vi "calc_VoltageStepWaveform_v0.03.vi"(0 "New input cluster":T1={"Which Position to use for Experiment"=enum."Jumper Safe Position", "Duration (s)"=0.0, "Delay (s)"=0.0, "Step Width (s)"=0.0, "Voltage Start (mV)"=1.0, "Voltage Step (mV)"=1.0, "Replicates"=1.0, "Voltage End (mV)"=0.0, "Number of Step"=0.0, "Vholding (mV)"=2.0, "Valve 1 Position"=2, "Valve 2 Position"=2, "Valve 3 Position"=2, "valve 1 used now?"=FALSE, "valve 2 used now?"=FALSE, "valve 3 used now? "=TRUE, "Total Step Time (s)"=0.0, "Maintain Final Voltage until end?"=TRUE, "protocol Preview"=[]} {"Valve 3 Position" min=1 max=8; "Valve 2 Position" min=1 max=8; "Valve 1 Position" min=1 max=8}, 1 "Clear Waveform?":bool, 5 "Old input cluster":T1={"Which Position to use for Experiment"=enum."Jumper Safe Position", "Duration (s)"=0.0, "Delay (s)"=0.0, "Step Width (s)"=0.0, "Voltage Start (mV)"=1.0, "Voltage Step (mV)"=1.0, "Replicates"=1.0, "Voltage End (mV)"=0.0, "Number of Step"=0.0, "Vholding (mV)"=2.0, "Valve 1 Position"=2, "Valve 2 Position"=2, "Valve 3 Position"=2, "valve 1 used now?"=FALSE, "valve 2 used now?"=FALSE, "valve 3 used now? "=TRUE, "Total Step Time (s)"=0.0, "Maintain Final Voltage until end?"=TRUE, "protocol Preview"=[]} {"Valve 3 Position" min=1 max=8; "Valve 2 Position" min=1 max=8; "Valve 1 Position" min=1 max=8}, 7 "sample freq":i32=10000, 11 "error in":errorcluster) -> (4 "output cluster":T1={"Which Position to use for Experiment"=enum."Jumper Safe Position", "Duration (s)"=0.0, "Delay (s)"=0.0, "Step Width (s)"=0.0, "Voltage Start (mV)"=1.0, "Voltage Step (mV)"=1.0, "Replicates"=1.0, "Voltage End (mV)"=0.0, "Number of Step"=0.0, "Vholding (mV)"=2.0, "Valve 1 Position"=2, "Valve 2 Position"=2, "Valve 3 Position"=2, "valve 1 used now?"=FALSE, "valve 2 used now?"=FALSE, "valve 3 used now? "=TRUE, "Total Step Time (s)"=0.0, "Maintain Final Voltage until end?"=TRUE, "protocol Preview"=[]} {"Valve 3 Position" min=1 max=8; "Valve 2 Position" min=1 max=8; "Valve 1 Position" min=1 max=8}, 15 "error out":errorcluster)   [LabVIEW 2019]
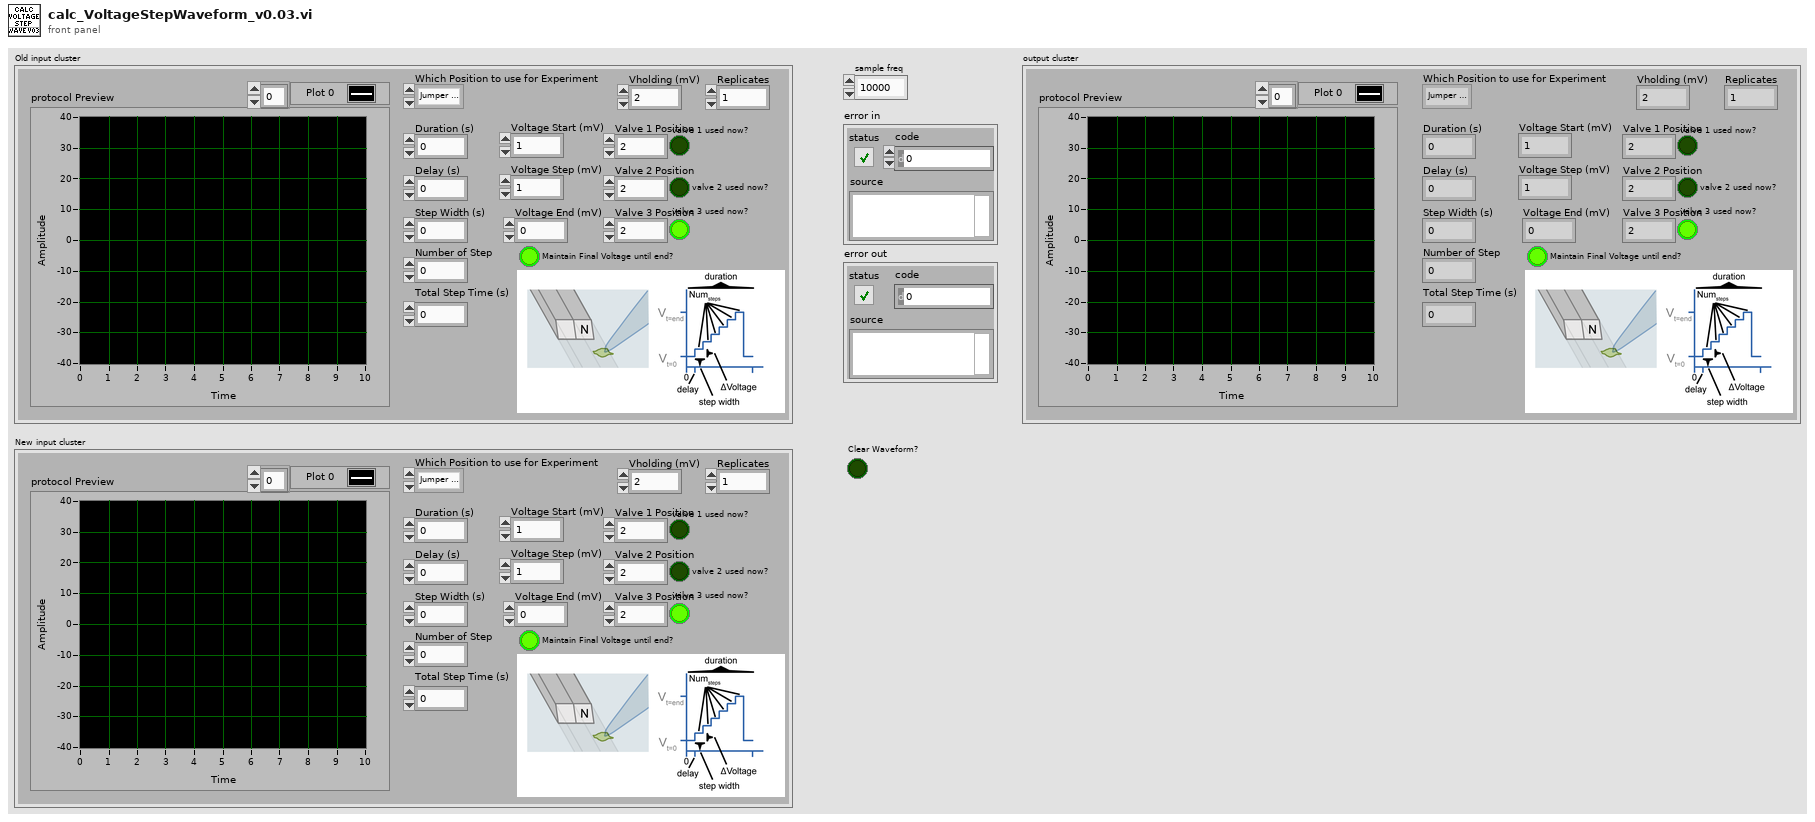
[diagram p1: front panel]
types:
  T1 = cluster{"Which Position to use for Experiment":enum16{"Jumper Safe Position", "Experiment Safe Position", "Jumper Position A", "Jumper Position B", "Jumper Position C", "Jumper Position o-A", "Jumper Position A-o", "Jumper Position A-B", "Jumper Position B-A", "Jumper Position B-C", "Jumper Position C-B", "Jumper Position C-o", "Jumper Position o-C", "Don't Move"}, "Duration (s)":dbl, "Delay (s)":dbl, "Step Width (s)":dbl, "Voltage Start (mV)":dbl, "Voltage Step (mV)":dbl, "Replicates":dbl, "Voltage End (mV)":dbl, "Number of Step":dbl, "Vholding (mV)":dbl, "Valve 1 Position":i16, "Valve 2 Position":i16, "Valve 3 Position":i16, "valve 1 used now?":bool, "valve 2 used now?":bool, "valve 3 used now? ":bool, "Total Step Time (s)":dbl, "Maintain Final Voltage until end?":bool, "protocol Preview":waveform(dbl)[]}
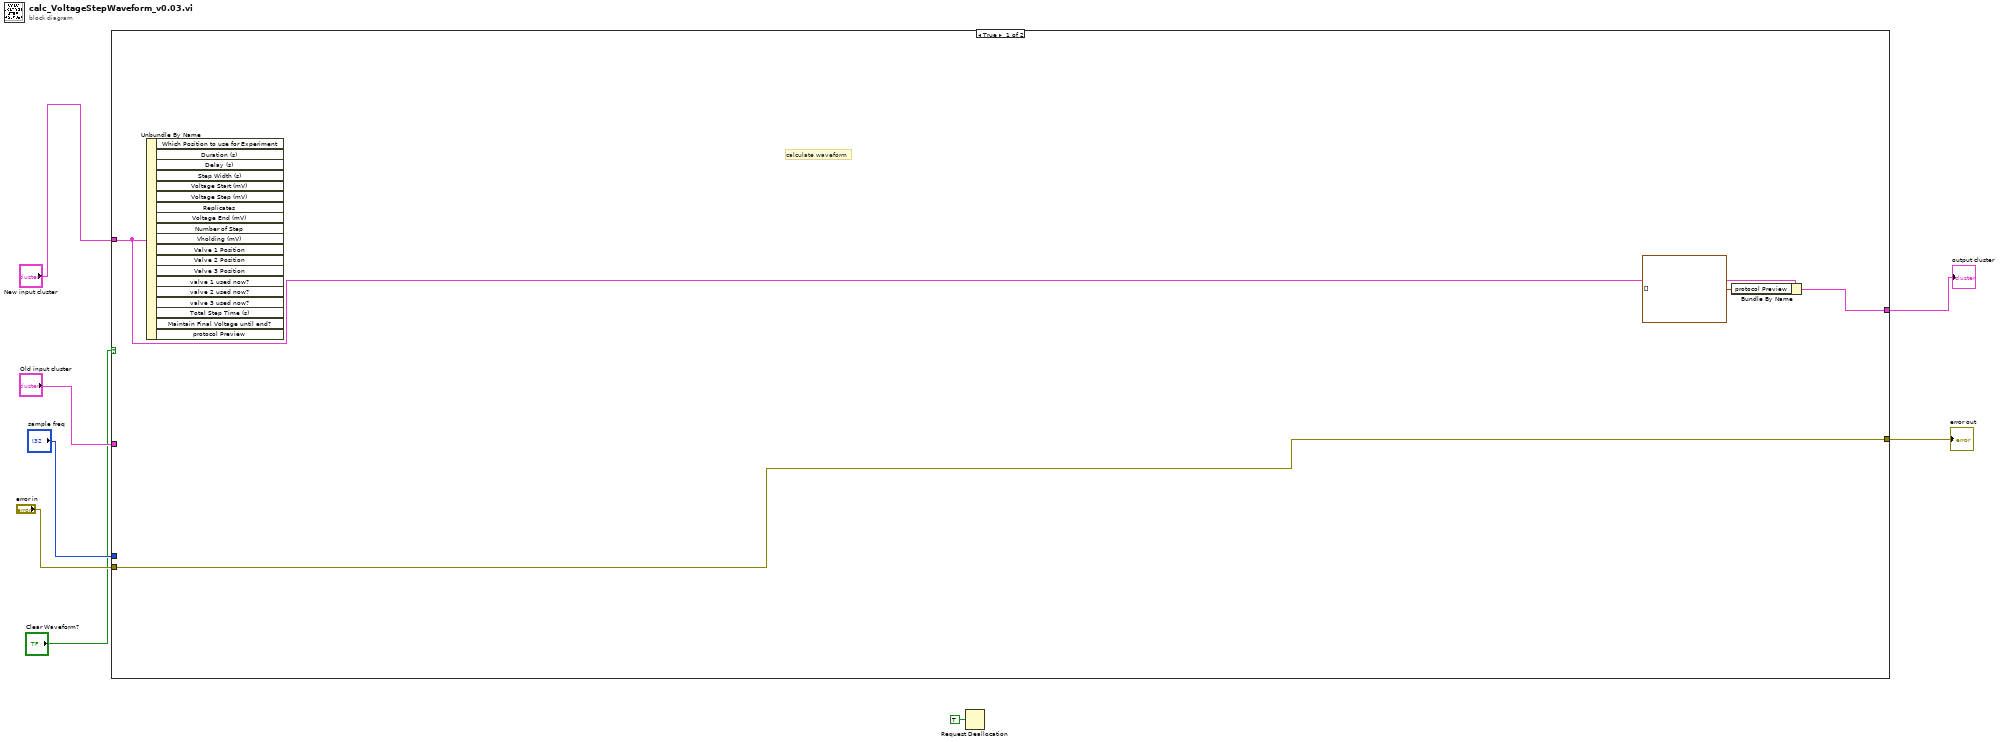
[diagram p0: block diagram]
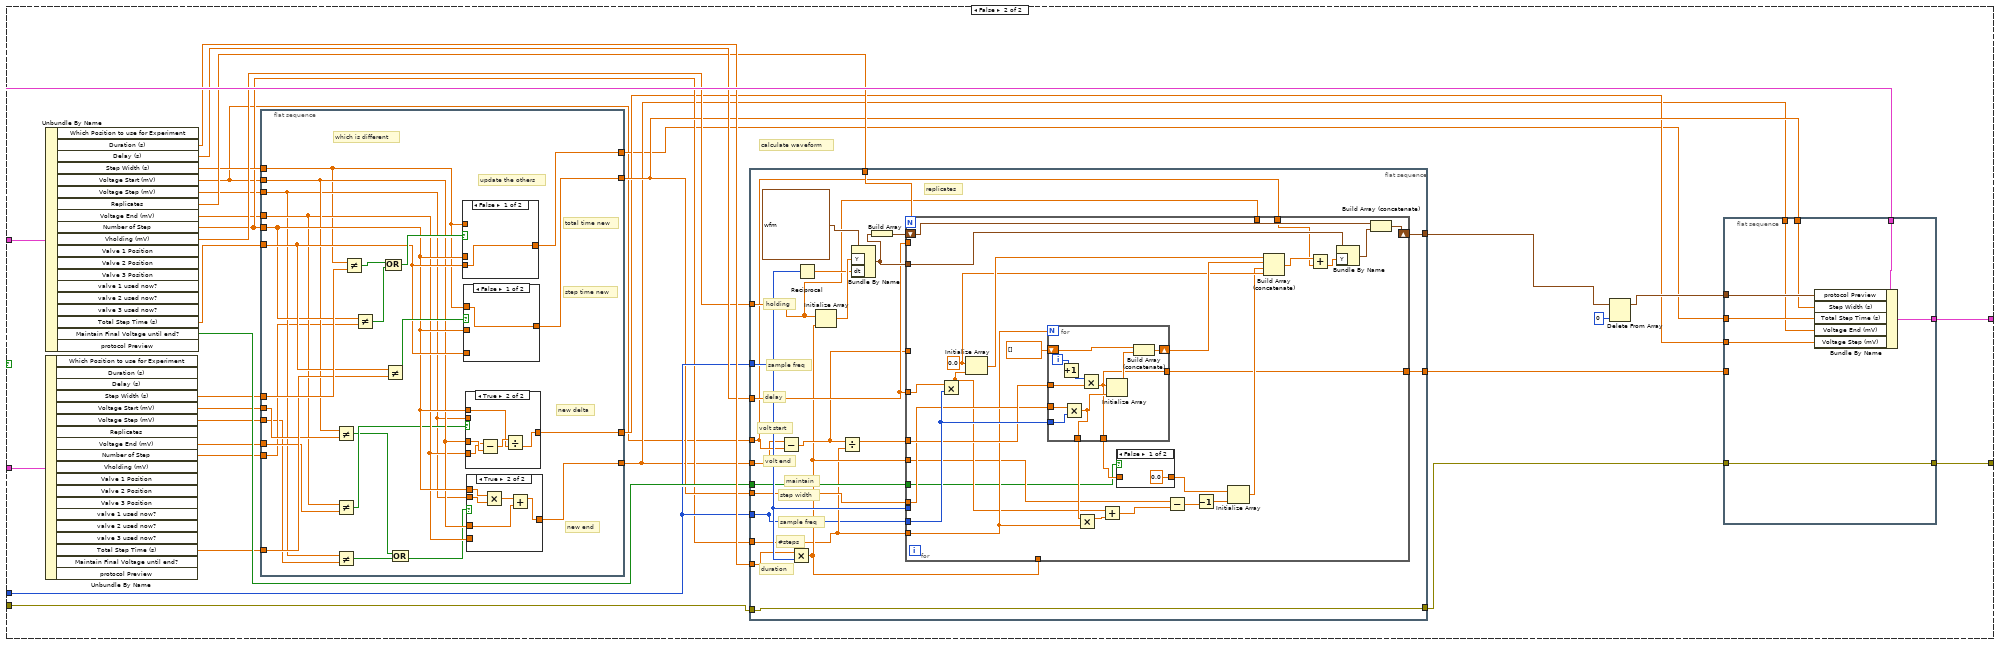
[diagram p2: hidden frame]
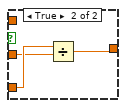
[diagram p5: hidden frame]
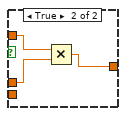
[diagram p6: hidden frame]
diagram:
  n1 = case shown="True" "Clear Waveform?" {
    tunnel: "New input cluster" -> [w12 w44]
    tunnel: [w11 w43] -> w7
    tunnel: "Old input cluster" -> [_ w42]
    tunnel: "error in" -> [w9 w38]
    tunnel: "sample freq" -> [_ w32]
    tunnel: [w9 w16] -> w3
    frame True {
      # "calculate waveform"
      n2 = Unbundle By Name(w12) -> ()  [unwired: 19 out]
      n3 = Bundle By Name(cluster=w12, "protocol Preview"=waveform(dbl)[] []) -> (w11:T1)
    }
    frame False {
      # "calculate waveform"
      n4 = Unbundle By Name(w42) -> ("Step Width (s)"=w31:dbl, "Voltage Start (mV)"=w25:dbl, "Voltage Step (mV)"=w13:dbl, "Voltage End (mV)"=w23:dbl, "Number of Step"=w19:dbl, "Total Step Time (s)"=w30:dbl)  [unwired: 13 out]
      n5 = Unbundle By Name(w44) -> ("Duration (s)"=w37:dbl, "Delay (s)"=w36:dbl, "Step Width (s)"=w29:dbl, "Voltage Start (mV)"=w14:dbl, "Voltage Step (mV)"=w22:dbl, "Replicates"=w35:dbl, "Voltage End (mV)"=w24:dbl, "Number of Step"=w26:dbl, "Vholding (mV)"=w34:dbl, "Total Step Time (s)"=w27:dbl, "Maintain Final Voltage until end?"=w33:bool)  [unwired: 8 out]
      n6 = flat-sequence {
        tunnel: w31 -> [w76]
        tunnel: w30 -> [w75]
        tunnel: w29 -> [w56]
        tunnel: [w73] -> w18
        tunnel: [w71] -> w28
        tunnel: w27 -> [w68]
        tunnel: w26 -> [w67]
        tunnel: w14 -> [w66]
        tunnel: w25 -> [w65]
        tunnel: w24 -> [w64]
        tunnel: w23 -> [w63]
        tunnel: w22 -> [w61]
        tunnel: [w59] -> w21
        tunnel: [w58] -> w20
        tunnel: w19 -> [w57]
        tunnel: w13 -> [w53]
        frame #0 {
          # "new end"
          # "new delta"
          # "step time new"
          # "total time new"
          # "update the others"
          # "which is different"
          n7 = Not Equal?(x=w66, y=w65) -> (x != y?=w54:bool)
          n8 = Not Equal?(x=w64, y=w63) -> (x != y?=w62:bool)
          n9 = Not Equal?(x=w61, y=w53) -> (x != y?=w60:bool)
          n10 = Not Equal?(x=w56, y=w76) -> (x != y?=w72:bool)
          n11 = Not Equal?(x=w67, y=w57) -> (x != y?=w69:bool)
          n12 = Not Equal?(x=w68, y=w75) -> (x != y?=w74:bool)
          n13 = Compound Arithmetic op=OR(w72, w69) -> (w70:bool)
          n14 = Compound Arithmetic op=OR(w54, w60) -> (w55:bool)
          n15 = case shown="False" w70 {
            tunnel: w56 -> [_ w96]
            tunnel: w67 -> [_ w95]
            tunnel: w68 -> [w93 _]
            tunnel: [w93 w94] -> w73
            frame False {
            }
            frame True {
              n16 = Multiply(x=w96, y=w95) -> (x*y=w94:dbl)
            }
          }
          n17 = case shown="False" w74 {
            tunnel: w56 -> [w89 _]
            tunnel: w67 -> [_ w91]
            tunnel: w68 -> [_ w92]
            tunnel: [w89 w90] -> w71
            frame False {
            }
            frame True {
              n18 = Divide(x=w92, y=w91) -> (x/y=w90:dbl)
            }
          }
          n19 = case shown="True" w62 {
            tunnel: w67 -> [_ w84]
            tunnel: w64 -> [_ w87]
            tunnel: w66 -> [_ w88]
            tunnel: w61 -> [w83 _]
            tunnel: [w83 w86] -> w59
            frame False {
            }
            frame True {
              n20 = Subtract(x=w87, y=w88) -> (x-y=w85:dbl)
              n21 = Divide(x=w85, y=w84) -> (x/y=w86:dbl)
            }
          }
          n22 = case shown="True" w55 {
            tunnel: w67 -> [_ w82]
            tunnel: w64 -> [w77 _]
            tunnel: w66 -> [_ w78]
            tunnel: w61 -> [_ w81]
            tunnel: [w77 w79] -> w58
            frame False {
            }
            frame True {
              n23 = Multiply(x=w82, y=w81) -> (x*y=w80:dbl)
              n24 = Add(x=w80, y=w78) -> (x+y=w79:dbl)
            }
          }
        }
      }
      n25 = flat-sequence {
        tunnel: w37 -> [w106]
        tunnel: [w98] -> _
        tunnel: w38 -> [w100]
        tunnel: w36 -> [w111]
        tunnel: w14 -> [w104]
        tunnel: w35 -> [w118]
        tunnel: w32 -> [w112]
        tunnel: w34 -> [w107]
        tunnel: w20 -> [w99]
        tunnel: w28 -> [w110]
        tunnel: w26 -> [w102]
        tunnel: w33 -> [w103]
        tunnel: [w101] -> w39
        tunnel: [w100] -> w17
        tunnel: [w99] -> _
        tunnel: w32 -> [w98]
        tunnel: [w97] -> w15
        frame #0 {
          # "replicates"
          # "duration"
          # "#steps"
          # "sample freq"
          # "step width"
          # "maintain"
          # "volt end"
          # "volt start"
          # "delay"
          # "sample freq"
          # "holding"
          n26 = Subtract(x=w99, y=w104) -> (x-y=w109:dbl)
          n27 = Multiply(x=w106, y=w112) -> (x*y=w105:dbl)
          n28 = Reciprocal(x=w112) -> (1/x=w108:dbl)
          n29 = Initialize Array(w107, w105) -> (w115:dbl[])
          n30 = Divide(x=w109, y=w102) -> (x/y=w113:dbl)
          n31 = Bundle By Name(cluster=waveform(dbl) {"t0"=timestamp(0 s since 1904-01-01), "dt"=1.0, "Y"=[]} ("signal out"), "Y"=w115, "dt"=w108) -> (w114:waveform(dbl))
          n32 = Build Array(w114) -> (w117:waveform(dbl)[])
          n33 = for {
            N: w118 -> [_]
            tunnel: w111 -> [_]
            shift-right: [w146] -> w101
            shift-left: w117 -> [w145]
            tunnel: w114 -> [w143]
            tunnel: w113 -> [w140]
            tunnel: w112 -> [_]
            tunnel: w111 -> [w136]
            tunnel: w110 -> [w135]
            tunnel: w109 -> [_]
            tunnel: w105 -> [_]
            tunnel: w107 -> [_]
            tunnel: w98 -> [w141]
            tunnel: w102 -> [w133]
            tunnel: w105 -> [w127]
            tunnel: w104 -> [w123]
            tunnel: w103 -> [w120]
            tunnel: [w119] -> w97
            w132 = 0.0 ("element")
            n34 = Multiply(x=w136, y=w141) -> (x*y=w128:dbl)
            n35 = Initialize Array(w132, w128) -> (w142:dbl[])
            n36 = for {
              N: w133 -> [_]
              tunnel: w135 -> [w157]
              tunnel: w141 -> [w156]
              tunnel: w140 -> [w155]
              shift-right: [w153] -> w139
              shift-left: dbl[] [] -> [w152]
              tunnel: [w149] -> w122
              tunnel: [w151] -> w129
              tunnel: [w149] -> w119
              i -> [w154]
              n37 = Increment(x=w154) -> (x+1=w150:i32)
              n38 = Multiply(x=w157, y=w156) -> (x*y=w151:dbl)
              n39 = Multiply(x=w150, y=w155) -> (x*y=w149:dbl)
              n40 = Initialize Array(w149, w151) -> (w158:dbl[])
              n41 = Build Array (concatenate)(w152, w158) -> (w153:dbl[])
            }
            n42 = Multiply(x=w129, y=w133) -> (x*y=w134:dbl)
            n43 = Add(x=w128, y=w134) -> (x+y=w137:dbl)
            n44 = case shown="False" w120 {
              tunnel: w122 -> [_ w148]
              tunnel: [0.0 w148] -> w121
              frame False {
              }
              frame True {
              }
            }
            n45 = Subtract(x=w127, y=w137) -> (x-y=w126:dbl)
            n46 = Decrement(x=w126) -> (x-1=w130:dbl)
            n47 = Initialize Array(w121, w130) -> (w131:dbl[])
            n48 = Build Array (concatenate)(w142, w139, w131, w132) -> (w124:dbl[])
            n49 = Add(x=w124, y=w123) -> (x+y=w125:dbl[])
            n50 = Bundle By Name(cluster=w143, "Y"=w125) -> (w144:waveform(dbl))
            n51 = Build Array (concatenate)(w145, w144) -> (w146:waveform(dbl)[])
          }
        }
      }
      n52 = Delete From Array(array=w39, index=0) -> (array with subset deleted=w40:waveform(dbl)[])  [unwired: 1 in, 1 out]
      n53 = flat-sequence {
        tunnel: w44 -> [w52]
        tunnel: [w51] -> w43
        tunnel: w40 -> [w50]
        tunnel: w28 -> [w49]
        tunnel: w21 -> [w48]
        tunnel: w20 -> [w45]
        tunnel: w18 -> [w47]
        tunnel: w17 -> [w46]
        tunnel: [w46] -> w16
        tunnel: w15 -> [_]
        frame #0 {
          n54 = Bundle By Name(cluster=w52, "protocol Preview"=w50, "Step Width (s)"=w49, "Total Step Time (s)"=w47, "Voltage End (mV)"=w45, "Voltage Step (mV)"=w48) -> (w51:T1)
        }
      }
    }
  }
  "output cluster" <- w7
  "error out" <- w3
  n55 = Request Deallocation(TRUE ("flag")) -> ()
